vi "Set Velocity Setpoint.vi"(8 "error in (no error)":errorcluster, 10 "ccw velocity (rpm)":dbl, 11 "KUKA youBot gripper motor in":refnum<class "NI_Robotics_KUKA youBot Gripper Motor.lvclass">) -> (0 "error out":errorcluster, 3 "KUKA youBot gripper motor out":refnum<class "NI_Robotics_KUKA youBot Gripper Motor.lvclass">)   [LabVIEW 2017, in "NI_Robotics_KUKA youBot Host.lvlib" / "NI_Robotics_KUKA youBot Gripper Motor.lvclass"]
uses:
  <vilib>/robotics/KUKA youBot/Motor/Gripper Motor/NI_Robotics_KUKA youBot Gripper Motor.lvclass
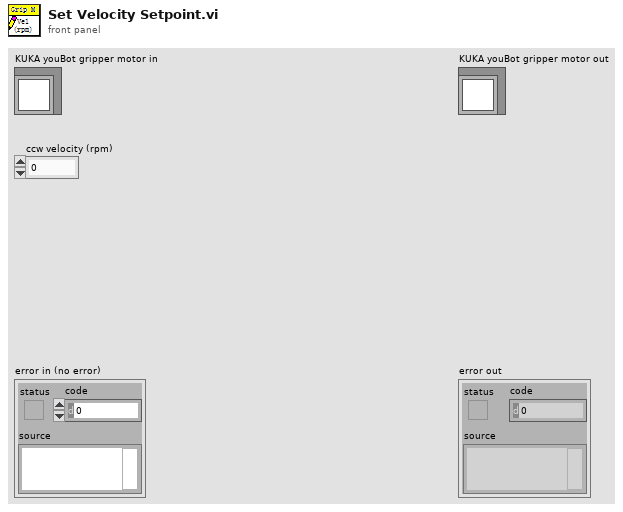
[diagram p1: front panel]
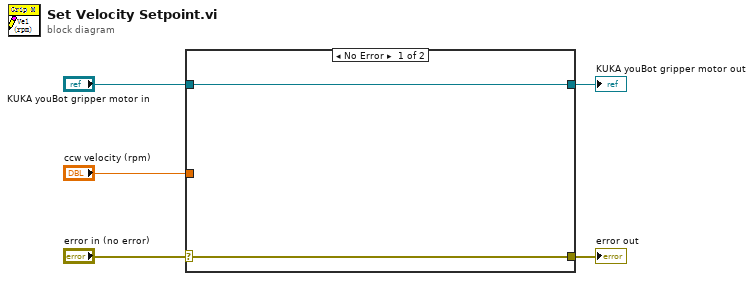
[diagram p0: block diagram]
diagram:
  n1 = case shown="No Error" "error in (no error)" {
    selector: "error in (no error)" -> [w7 w8]
    tunnel: [w7 w8] -> w4
    tunnel: [w6 w9] -> w2
    tunnel: "KUKA youBot gripper motor in" -> [w6 w9]
    tunnel: "ccw velocity (rpm)" -> [_ _]
    frame No Error {
    }
    frame Error {
    }
  }
  "error out" <- w4
  "KUKA youBot gripper motor out" <- w2
